vi "HB_ServeByBuffer.vi"() -> ()   [LabVIEW 2009, in "HB_DIM_Examples.lvlib"]
doc: "This VI implements a DIM server, that publishes a loop counter as a DIM service"
uses:
  HB_DIM_Examples.lvlib
  lib.lib/DimLVEvent/LVDimInterface/LVDimInterface.lvlib
panel:
  out "error out":errorcluster
  in  "update interval [ms]":u32=1000
  out "loopCounter":i32
  in  "stop":bool
  in  "serviceName":string="HB_Simple_0_y"
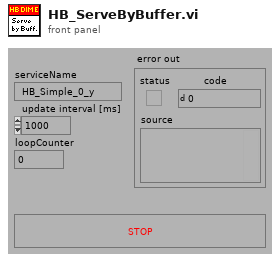
[diagram p1: front panel]
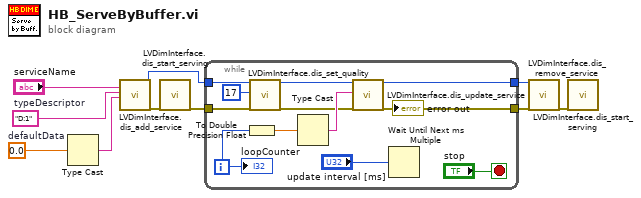
[diagram p0: block diagram]
diagram:
  w6 = 0.0  # defaultData
  w3 = "D:1"  # typeDescriptor
  n1 = Type Cast(x=w6) -> (*(type *) &x=w5:string)  [unwired: 1 out]
  n2 = call "LVDimInterface.dis_add_service.vi"("serviceName"="serviceName", "typeDescriptor"=w3, "data"=w5) -> ("my_serviceID"=w2:i32, "error out"=w9:errorcluster)  [unwired: 2 in, 13 out]
  n3 = call "LVDimInterface.dis_start_serving.vi"("error in (no error)"=w9) -> ("error out"=w8:errorcluster)  [unwired: 1 in, 17 out]
  n4 = while {
    tunnel: [w20] -> w10
    tunnel: w8 -> [w18]
    tunnel: [w11] -> w7
    tunnel: w2 -> [w15]
    i -> [w19]
    stop <- "stop" stop-if-true
    n5 = To Double Precision Float(number=w19) -> (double precision float=w12:dbl)
    n6 = call "LVDimInterface.dis_set_quality.vi"("my_serviceID"=w15, "quality"=17, "error in (no error)"=w18) -> ("my_serviceID (out)"=w14:i32, "error out"=w13:errorcluster)  [unwired: 15 out]
    n7 = Type Cast(x=w12) -> (*(type *) &x=w17:string)  [unwired: 1 out]
    n8 = call "LVDimInterface.dis_update_service.vi"("my_serviceID"=w14, "data"=w17, "error in (no error)"=w13) -> ("my_serviceID out"=w20:i32, "error out"=w11:errorcluster)  [unwired: 2 in, 13 out]
    "error out" <- w11
    n9 = Wait Until Next ms Multiple(millisecond multiple="update interval [ms]") -> ()  [unwired: 1 out]
    "loopCounter" <- w19
  }
  n10 = call "LVDimInterface.dis_remove_service.vi"("my_serviceID"=w10, "error in (no error)"=w7) -> ("error out"=w1:errorcluster)  [unwired: 1 in, 16 out]
  n11 = call "LVDimInterface.dis_start_serving.vi"("error in (no error)"=w1) -> ()  [unwired: 1 in, 18 out]
